vi "readUTC.vi"(2 "error out 2":errorcluster, 3 "gps handle":refnum<k15>) -> (0 "error out":errorcluster, 1 "time":timestamp)   [LabVIEW 2010]
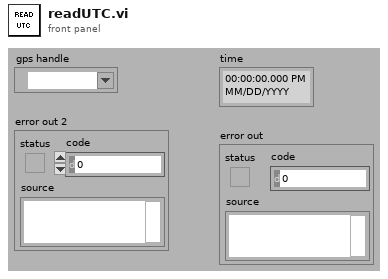
[diagram p1: front panel]
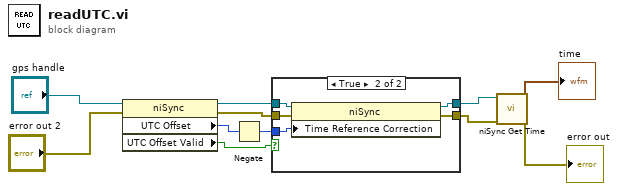
[diagram p0: block diagram]
diagram:
  n1 = property class="niSync"(reference="gps handle", error in="error out 2") -> (reference out=w6:refnum<k15>, error out=w5:errorcluster, "UTC Offset"=w4:i32, "UTC Offset Valid"=w7:bool)
  n2 = Negate(x=w4) -> (-x=w3:i32)
  n3 = case shown="True" w7 {
    tunnel: w6 -> [w13 w18]
    tunnel: w5 -> [w12 w17]
    tunnel: [w13 w16] -> w2
    tunnel: [w12 w15] -> w1
    tunnel: w3 -> [_ w14]
    frame False {
    }
    frame True {
      n4 = property class="niSync"(reference=w18, error in=w17, "Time Reference Correction"=w14) -> (reference out=w16:refnum<k15>, error out=w15:errorcluster)
    }
  }
  n5 = call <instrlib>:"niSync Get Time.vi"("error in (no error)"=w1, "instrument handle"=w2) -> ("error out"=→"error out":errorcluster, "time"=→"time":timestamp)  [unwired: 5 in, 1 out]
